vi "AlazarSetTriggerTimeOut.vi"(8 "error in (no error)":errorcluster, 10 "Timeout Ticks":u32, 11 "Handle":u32) -> (0 "error out":errorcluster, 2 "Return Code":u32, 3 "Handle":u32)   [LabVIEW 2018]
doc: "Set the time to wait for a trigger event before automatically generating a trigger event."
uses:
  ATSApi.dll
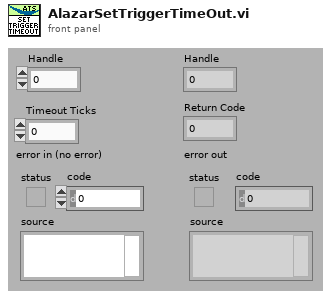
[diagram p1: front panel]
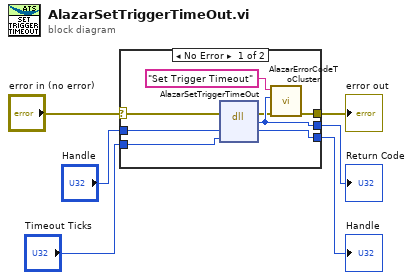
[diagram p0: block diagram]
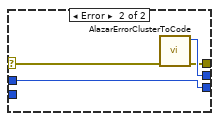
[diagram p2: hidden frame]
diagram:
  n1 = case shown="No Error" "error in (no error)" {
    selector: "error in (no error)" -> [w8 w18]
    tunnel: [w11 w15] -> w5
    tunnel: [w13 w17] -> w4
    tunnel: "Handle" -> [w14 w16]
    tunnel: [w10 w16] -> w2
    tunnel: "Timeout Ticks" -> [w9 _]
    frame No Error {
      n2 = dll-call lib="ATSApi.dll" fn="AlazarSetTriggerTimeOut"(error in=w8, "handle"=w14, "timeoutTicks"=w9) -> (error out=w7:errorcluster, "return type"=w13:u32, "handle"=w10:u32)  [unwired: 3 in, 1 out]
      n3 = call "AlazarErrorCodeToCluster.vi"("error in (no error)"=w7, "Error Code In"=w13, "Message"="Set Trigger Timeout") -> ("error out"=w11:errorcluster)  [unwired: 7 in, 1 out]
    }
    frame Error {
      n4 = call "AlazarErrorClusterToCode.vi"("error in (no error)"=w18) -> ("error out"=w15:errorcluster, "Error Code"=w17:u32)  [unwired: 9 in]
    }
  }
  "Handle" <- w2
  "error out" <- w5
  "Return Code" <- w4
